vi "CMN_DescribeDriverErrors.vi"(0 "message":string, 2 "OK message":string="DONE", 3 "error in (no error)":errorcluster, 5 "database name":string="DBS") -> (7 "error?":bool, 8 "astroerrors":string, 10 "error out":errorcluster)   [LabVIEW 2016]
doc: "This subVI tests the error status output of one or more low-level functions or subVIs that output a numeric error code, and creates an error out cluster that can be wired to the Simple or General Error Handler in order to identify the error and describe it to the user.\n\nThe error in cluster is tested first. If error? is no-error, the elements of the error codes array are tested next for non-zero values. The first error found terminates the test, and error out identifies that error. Use a Build Array function to assemble the individual error codes.\n\nYou can optionally use the source messages string to pass on the source of the error. Enter one line of text for each element of the error codes array. \n\nThe error? status is TRUE on any error."
uses:
  DBSHAND/private/vis/DatabaseHand_Element_Get(string).vi
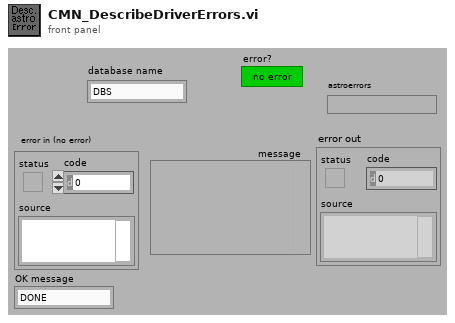
[diagram p1: front panel]
types:
  T1 = typedef "DatabaseHand_RefNum.ctl" = refnum<vi>
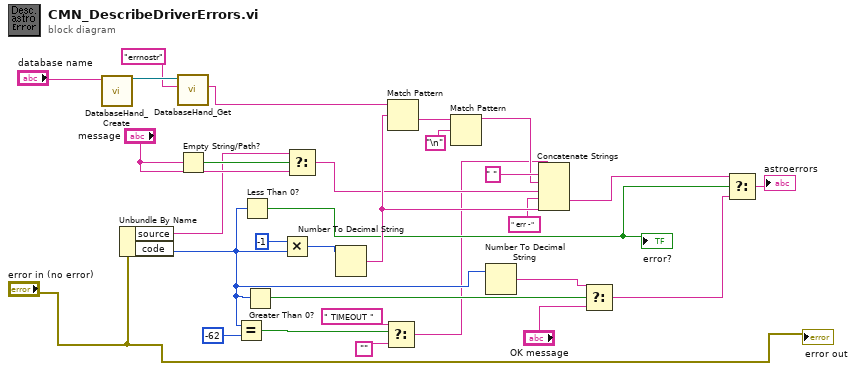
[diagram p0: block diagram]
diagram:
  n1 = call "DatabaseHand_Create.vi"("Name"="database name") -> ("Database RefNum out"=w3:T1)  [unwired: 1 in, 9 out]
  n2 = Unbundle By Name("error in (no error)") -> ("source"=w18:string, "code"=w12:i32)
  n3 = call-poly "DatabaseHand_Get.vi"("name"="errnostr", "Database RefNum in"=w3) -> ("value"=w2:string)  [unwired: 3 in, 6 out]
  n4 = Empty String/Path?(string/path="message") -> (empty?=w20:bool)
  n5 = Equal?(x=w12, y=-62) -> (x = y?=w10:bool)
  n6 = Less Than 0?(x=w12) -> (x < 0?=w22:bool)
  "error?" <- w22
  n7 = Greater Than 0?(x=w12) -> (x > 0?=w15:bool)
  n8 = Multiply(x=-1, y=w12) -> (x*y=w24:i32)
  n9 = Select(t=w18, s=w20, f="message") -> (s? t:f=w17:string)
  n10 = Number To Decimal String(number=w24) -> (decimal integer string=w26:string)  [unwired: 1 out]
  n11 = Select(t=" TIMEOUT ", s=w10, f="") -> (s? t:f=w7:string)
  n12 = Match Pattern(string=w2, regular expression=w26) -> (after substring=w28:string)  [unwired: 4 out]
  n13 = Match Pattern(string=w28, regular expression="\n") -> (before substring=w16:string)  [unwired: 4 out]
  n14 = Number To Decimal String(number=w12) -> (decimal integer string=w13:string)  [unwired: 1 out]
  n15 = Concatenate Strings(w7, " ", w16, w17, " err -", w26) -> (w30:string)
  n16 = Select(t=w13, s=w15, f="OK message") -> (s? t:f=w14:string)
  n17 = Select(t=w30, s=w22, f=w14) -> (s? t:f=→"astroerrors":string)
  "error out" <- "error in (no error)"
